vi "Lunar PNSN encode_decode.vi"(8 "Lunar PN Frame In":T3, 9 "Lunar SN Frame In":T4, 10 "Lunar PN In":T1, 11 "Lunar SN In":T2) -> (0 "Lunar PN Out":T1, 1 "Lunar SN Out":T2, 2 "Lunar PN Frame Out":T3, 3 "Lunar SN Frame Out":T4)   [LabVIEW 2021]
uses:
  LunarPN.ctl
  LunarSN Frame.ctl
  LunarPN Frame.ctl
  LunarSN.ctl
panel:
  # "-"
  # "-"
  # "-"
  # "-"
  # "-"
  # "-"
  # "-"
  # "-"
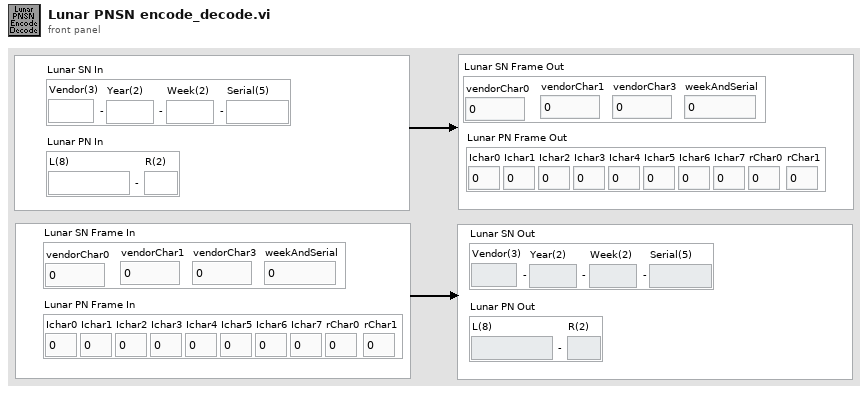
[diagram p1: front panel]
types:
  T1 = typedef "LunarPN.ctl" = cluster{"L(8)":string, "R(2)":string}
  T2 = typedef "LunarSN.ctl" = cluster{"Vendor(3)":string, "Year(2)":string, "Week(2)":string, "Serial(5)":string}
  T3 = typedef "LunarPN Frame.ctl" = cluster{"Ichar0":u8, "Ichar1":u8, "Ichar2":u8, "Ichar3":u8, "Ichar4":u8, "Ichar5":u8, "Ichar6":u8, "Ichar7":u8, "rChar0":u8, "rChar1":u8}
  T4 = typedef "LunarSN Frame.ctl" = cluster{"vendorChar0":u8, "vendorChar1":u8, "vendorChar3":u8, "weekAndSerial":u32}
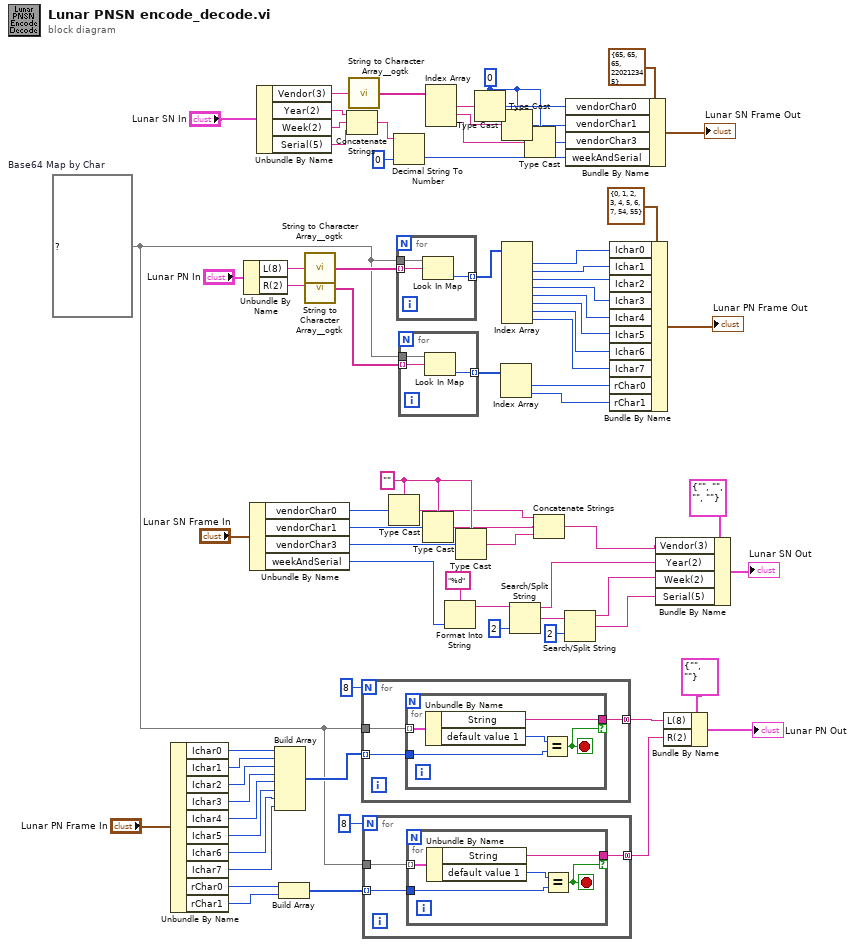
[diagram p0: block diagram]
diagram:
  w38 = "" ("element")
  w3 = map{string, u8} {"+"=62, "/"=63, "0"=52, "1"=53, "2"=54, "3"=55, "4"=56, "5"=57, "6"=58, "7"=59, "8"=60, "9"=61, "A"=0, "B"=1, "C"=2, "D"=3, "E"=4, "F"=5, "G"=6, "H"=7, "I"=8, "J"=9, "K"=10, "L"=11, "M"=12, "N"=13, "O"=14, "P"=15, "Q"=16, "R"=17, "S"=18, "T"=19, "U"=20, "V"=21, "W"=22, "X"=23, "Y"=24, "Z"=25, "a"=26, "b"=27, "c"=28, "d"=29, "e"=30, "f"=31, "g"=32, "h"=33, "i"=34, "j"=35, "k"=36, "l"=37, "m"=38, "n"=39, "o"=40, "p"=41, "q"=42, "r"=43, "s"=44, "t"=45, "u"=46, "v"=47, "w"=48, "x"=49, "y"=50, "z"=51}  # Base64 Map by Char
  w71 = u8 0 ("vendorChar0")
  n1 = Unbundle By Name("Lunar PN Frame In") -> ("Ichar0"=w16:u8, "Ichar1"=w15:u8, "Ichar2"=w14:u8, "Ichar3"=w13:u8, "Ichar4"=w12:u8, "Ichar5"=w11:u8, "Ichar6"=w10:u8, "Ichar7"=w9:u8, "rChar0"=w7:u8, "rChar1"=w6:u8)
  n2 = Unbundle By Name("Lunar PN In") -> ("L(8)"=w60:string, "R(2)"=w59:string)
  n3 = Unbundle By Name("Lunar SN Frame In") -> ("vendorChar0"=w39:u8, "vendorChar1"=w37:u8, "vendorChar3"=w36:u8, "weekAndSerial"=w35:u32)
  n4 = Unbundle By Name("Lunar SN In") -> ("Vendor(3)"=w77:string, "Year(2)"=w67:string, "Week(2)"=w66:string, "Serial(5)"=w65:string)
  n5 = Build Array(w16, w15, w14, w13, w12, w11, w10, w9) -> (w17:u8[])
  n6 = Build Array(w7, w6) -> (w8:u8[])
  n7 = call <userlib>:"String to Character Array__ogtk.vi"("Input String"=w60) -> ("Character Array"=w58:string[])
  n8 = call <userlib>:"String to Character Array__ogtk.vi"("Input String"=w59) -> ("Character Array"=w57:string[])
  n9 = Concatenate Strings(w67, w66, w65) -> (w64:string)
  n10 = call <userlib>:"String to Character Array__ogtk.vi"("Input String"=w77) -> ("Character Array"=w76:string[])
  n11 = for {
    N: 8 -> [_]
    tunnel: w3 -> [w80]
    tunnel: w17 -> [w79] mode=indexing
    tunnel: [w78] -> w20 mode=concatenating
    n12 = for {
      tunnel: w80 -> [w85] mode=indexing
      tunnel: w79 -> [w83]
      tunnel: [w82] -> w78 if=w81
      stop <- w81 stop-if-true
      n13 = Unbundle By Name(w85) -> ("String"=w82:string, "default value 1"=w84:u8)
      n14 = Equal?(x=w84, y=w83) -> (x = y?=w81:bool)
    }
  }
  n15 = for {
    N: 8 -> [_]
    tunnel: w3 -> [w88]
    tunnel: w8 -> [w87] mode=indexing
    tunnel: [w86] -> w5 mode=concatenating
    n16 = for {
      tunnel: w88 -> [w93] mode=indexing
      tunnel: w87 -> [w91]
      tunnel: [w90] -> w86 if=w89
      stop <- w89 stop-if-true
      n17 = Unbundle By Name(w93) -> ("String"=w90:string, "default value 1"=w92:u8)
      n18 = Equal?(x=w92, y=w91) -> (x = y?=w89:bool)
    }
  }
  n19 = Type Cast(type=w38, x=w39) -> (*(type *) &x=w29:string)
  n20 = Decimal String To Number(string=w64, default (0L)=u32 0 ("default (0 I32)")) -> (number=w62:u32)  [unwired: 1 in, 1 out]
  n21 = for {
    tunnel: w3 -> [w96]
    tunnel: w58 -> [w95] mode=indexing
    tunnel: [w94] -> w56 mode=indexing
    n22 = Look In Map(map=w96, key=w95) -> (value=w94:u8)  [unwired: 1 in, 1 out]
  }
  n23 = for {
    tunnel: w3 -> [w99]
    tunnel: w57 -> [w98] mode=indexing
    tunnel: [w97] -> w47 mode=indexing
    n24 = Look In Map(map=w99, key=w98) -> (value=w97:u8)  [unwired: 1 in, 1 out]
  }
  n25 = Type Cast(type=w38, x=w37) -> (*(type *) &x=w28:string)
  n26 = Index Array(array=w76) -> (element #1=w75:string, element #2=w73:string, element #3=w72:string)  [unwired: 3 in]
  n27 = Format Into String(format string="%d", w35) -> (resulting string=w33:string)  [unwired: 2 in, 1 out]
  n28 = Type Cast(type=w38, x=w36) -> (*(type *) &x=w27:string)
  n29 = Type Cast(type=w71, x=w75) -> (*(type *) &x=w74:u8)
  n30 = Index Array(array=w47) -> (element #1=w46:u8, element #2=w45:u8)  [unwired: 2 in]
  n31 = Type Cast(type=w71, x=w73) -> (*(type *) &x=w70:u8)
  n32 = Index Array(array=w56) -> (element #1=w55:u8, element #2=w54:u8, element #3=w53:u8, element #4=w52:u8, element #5=w51:u8, element #6=w50:u8, element #7=w49:u8, element #8=w48:u8)  [unwired: 8 in]
  n33 = Search/Split String(string=w33, offset (0)=2) -> (substring before match=w25:string, match + rest of string=w24:string)  [unwired: 1 in, 1 out]
  n34 = Type Cast(type=w71, x=w72) -> (*(type *) &x=w69:u8)
  n35 = Concatenate Strings(w29, w28, w27) -> (w26:string)
  n36 = Search/Split String(string=w24, offset (0)=2) -> (substring before match=w23:string, match + rest of string=w22:string)  [unwired: 1 in, 1 out]
  n37 = Bundle By Name(cluster=T4 {"vendorChar0"=65, "vendorChar1"=65, "vendorChar3"=65, "weekAndSerial"=220212345} ("Lunar SN Frame"), "vendorChar0"=w74, "vendorChar1"=w70, "vendorChar3"=w69, "weekAndSerial"=w62) -> (→"Lunar SN Frame Out":T4)
  n38 = Bundle By Name(cluster=T3 {"Ichar0"=0, "Ichar1"=1, "Ichar2"=2, "Ichar3"=3, "Ichar4"=4, "Ichar5"=5, "Ichar6"=6, "Ichar7"=7, "rChar0"=54, "rChar1"=55} ("Lunar PN Frame"), "Ichar0"=w55, "Ichar1"=w54, "Ichar2"=w53, "Ichar3"=w52, "Ichar4"=w51, "Ichar5"=w50, "Ichar6"=w49, "Ichar7"=w48, "rChar0"=w46, "rChar1"=w45) -> (→"Lunar PN Frame Out":T3)
  n39 = Bundle By Name(cluster=T2 {"Vendor(3)"="", "Year(2)"="", "Week(2)"="", "Serial(5)"=""} ("Lunar SN Out"), "Vendor(3)"=w26, "Year(2)"=w25, "Week(2)"=w23, "Serial(5)"=w22) -> (→"Lunar SN Out":T2)
  n40 = Bundle By Name(cluster=T1 {"L(8)"="", "R(2)"=""} ("Lunar PN Out"), "L(8)"=w20, "R(2)"=w5) -> (→"Lunar PN Out":T1)
